vi "Untitled 3.vi"() -> ()   [LabVIEW 2019]
panel:
  in  "Array":u32[](array[colorbox])
  out "Color Box":u32(colorbox)
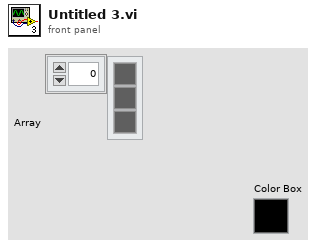
[diagram p1: front panel]
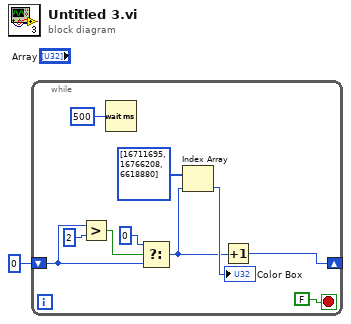
[diagram p0: block diagram]
diagram:
  n1 = while {
    shift-right: [w6] -> _
    shift-left: 0 -> [w3]
    stop <- FALSE stop-if-true
    n2 = Greater?(x=w3, y=2) -> (0:w4:bool)
    n3 = Wait (ms)(milliseconds to wait=u32 500) -> ()  [unwired: 1 out]
    n4 = Select(t=0, s=w4, f=w3) -> (s? t:f=w5:i32)
    n5 = Index Array(array=u32[] [16711695, 16766208, 6618880] ("Array 2"), index=w5) -> (element=→"Color Box":u32)
    n6 = Increment(x=w5) -> (x+1=w6:i32)
  }
